vi "niDTS WLAN VHT Rx Test Initialize.vi"(0 "Dut Reference":T2, 5 "SystemTechnologyCatalog":refnum<class "niDTS SystemTechnologyCatalog.lvclass">, 7 "SystemDut":refnum<class "niDTS SystemDut.lvclass">, 9 "Logger Reference":T1, 11 "error in (no error)":errorcluster) -> (4 "Dummy Test Handle out":T3, 6 "AllowAsync":bool=TRUE, 15 "error out":errorcluster)   [LabVIEW 2014, in "niDTS WLAN.lvlib"]
uses:
  niDTS WLAN.lvlib
  Rx Test/Includes/niDTS WLAN Rx Test INC Handle.ctl
  Rx Test/Objects/BASE_class/niDTS WLAN Rx Test.lvclass
  Framework/Dut/Includes/niDTS Dut INC Handle.ctl
  Framework/Dut/Objects/BASE_class/niDTS Dut.lvclass
  Framework/Logger/Includes/niDTS Logger INC Handle.ctl
  Framework/Logger/Objects/BASE_class/niDTS Logger.lvclass
  TestStand/Station/Objects/SystemDut/niDTS SystemDut.lvclass
  TestStand/Station/Objects/SystemTechnologyCatalog/niDTS SystemTechnologyCatalog.lvclass
  Includes/niDTS WLAN INC Standard.ctl
  TestStand/niDTS TestStand.lvlib
  Framework/niDTS Framework.lvlib
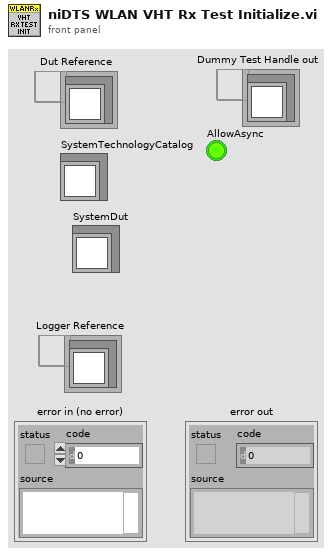
[diagram p1: front panel]
types:
  T1 = typedef "niDTS Framework.lvlib/niDTS Logger INC Handle.ctl" = refnum<data-value>
  T2 = typedef "niDTS Framework.lvlib/niDTS Dut INC Handle.ctl" = refnum<data-value>
  T3 = typedef "niDTS WLAN.lvlib/niDTS WLAN Rx Test INC Handle.ctl" = refnum<data-value>
  T4 = typedef "niDTS WLAN.lvlib/niDTS WLAN INC Standard.ctl" = enum16{"802.11 b DSSS", "802.11 a/g OFDM", "802.11 n HT", "802.11 ac VHT"}
  T5 = typedef "niDTS TestStand.lvlib/niDTS TestStep INC Handle.ctl" = refnum<data-value>
  T6 = typedef "niDTS WLAN.lvlib/niDTS WLAN Rx Test INC Parameters.ctl" = cluster{"Standard":T4, "DSSS Data Rate (Mbps)":T7, "OFDM Data Rate (Mbps)":T8, "MCS Index":i32, "N Spatial Streams":i32, "Chains":bool[], "Bandwidth (Hz)":T9, "Channel":i32, "Power (dBm)":dbl, "Guard Interval":T10, "FEC Coding":T11, "16 symbols":bool, "Payload Length (bytes)":i32, "Idle Interval (s)":dbl, "External Attenuation (dB)":dbl[], "RX Measurement Parameters":T12}
  T7 = typedef "niDTS WLAN.lvlib/niDTS WLAN INC DSSS Data Rate.ctl" = enum16{"1", "2", "5.5", "11"}
  T8 = typedef "niDTS WLAN.lvlib/niDTS WLAN INC OFDM Data Rate.ctl" = enum16{"6", "9", "12", "18", "24", "36", "48", "54"}
  T9 = typedef "niDTS WLAN.lvlib/niDTS WLAN INC CH BW.ctl" = enum16{"20 MHz", "40 MHz", "80 MHz", "160 MHz"}
  T10 = typedef "niDTS WLAN.lvlib/niDTS WLAN INC GI.ctl" = enum16{"LONG", "SHORT"}
  T11 = typedef "niDTS WLAN.lvlib/niDTS WLAN INC FEC Coding.ctl" = enum16{"BCC", "LDPC"}
  T12 = typedef "niDTS WLAN.lvlib/niDTS WLAN INC RX Measurement Parameters.ctl" = cluster{"Number of Packets":i32, "MacAddress":string}
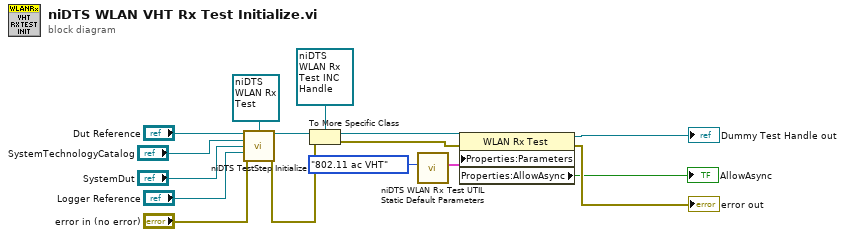
[diagram p0: block diagram]
diagram:
  n1 = call "niDTS TestStep Initialize.vi"("Dut Handle"="Dut Reference", "Test Type"=refnum<class "niDTS WLAN Rx Test.lvclass"> refnum ("Dummy Test.lvlib:Dummy Test.lvclass"), "SystemTechnologyCatalog"="SystemTechnologyCatalog", "SystemDut"="SystemDut", "Logger Reference"="Logger Reference", "error in (no error)"="error in (no error)") -> ("Test Handle out"=w14:T5, "error out"=w13:errorcluster)  [unwired: 8 in]
  n2 = To More Specific Class(target class=T3 refnum ("Dummy Test Handle"), reference=w14, error in=w13) -> (specific class reference=w7:T3, error out=w6:errorcluster)
  n3 = call "niDTS WLAN Rx Test UTIL Static Default Parameters.vi"("Standard"=niDTS_WLAN_INC_Standard."802.11 ac VHT") -> ("Static Default Parameters"=w8:T6)  [unwired: 10 in]
  n4 = property class="WLAN Rx Test"(reference=w7, error in=w6, "Properties:Parameters"=w8) -> (reference out=→"Dummy Test Handle out":T3, error out=→"error out":errorcluster, "Properties:AllowAsync"=→"AllowAsync":bool)
